vi "Get Parameters Configuration File Path.vi"(8 "error in":errorcluster, 11 "custom device ref":T1 format="%.0x") -> (0 "error out":errorcluster, 1 "MD5 checksum":string, 2 "parameters configuration file path":path, 3 "custom device ref out":T1 format="%.0x")   [LabVIEW 2024, in "AIM ARINC 429 Scripting.lvlib"]
doc: "Returns the <b>parameters configuration file path</b>. Systems configured in System Explorer must have a parameters configuration file. Scripted configurations do not require a parameters configuration file."
uses:
  AIM ARINC 429 Scripting.lvlib
  <vilib>/NI VeriStand/Custom Device API/Custom Device Item Ref.ctl
  Constants.vi
  <vilib>/NI VeriStand/Custom Device API/Get Item Property (Dependent File).vi
  <vilib>/NI VeriStand/Custom Device API/Custom Device API.lvlib
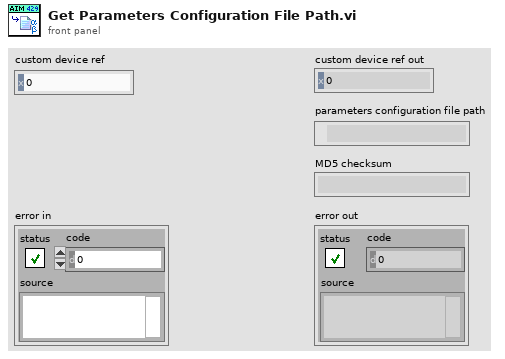
[diagram p1: front panel]
types:
  T1 = typedef "Custom Device API.lvlib/Custom Device Item Ref.ctl" = u64
  T2 = typedef "Custom Device API.lvlib/Dependent File Optional Info.ctl" = cluster{"Version":string, "RTDestination":path, "ForceDownload":bool, "SupportedTarget":string, "MD5":string}
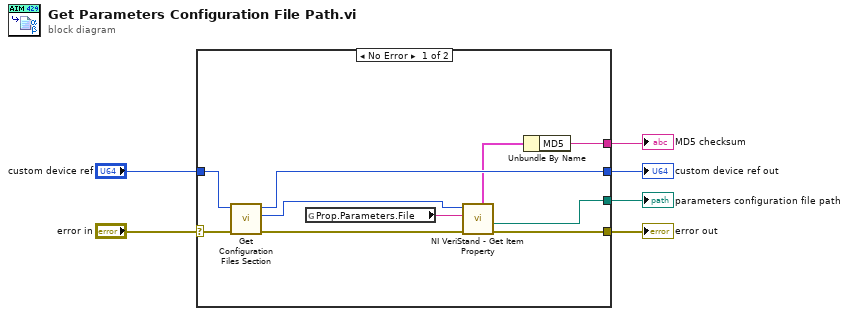
[diagram p0: block diagram]
diagram:
  n1 = case shown="No Error" "error in" {
    selector: "error in" -> [w11 w18]
    tunnel: "custom device ref" -> [w12 w17]
    tunnel: [w14 w18] -> w5
    tunnel: [w9 w17] -> w3
    tunnel: [w15 _] -> w2
    tunnel: [w7 _] -> w1
    frame No Error {
      n2 = call "Get Configuration Files Section.vi"("error in"=w11, "custom device ref"=w12) -> ("error out"=w10:errorcluster, "configuration files ref"=w13:T1, "custom device ref out"=w9:T1)  [unwired: 7 in]
      n3 = global read "Constants.vi" "Prop.Parameters.File"() -> (w16:string)
      n4 = call-poly <vilib>:"NI VeriStand - Get Item Property.vi"("error in (no error)"=w10, "Property Name"=w16, "Item Ref in"=w13) -> ("error out"=w14:errorcluster, "Path"=w15:path, "OptionalInfo"=w8:T2)  [unwired: 4 in, 2 out]
      n5 = Unbundle By Name(w8) -> ("MD5"=w7:string)
    }
    frame Error {
    }
  }
  "error out" <- w5
  "parameters configuration file path" <- w2
  "custom device ref out" <- w3
  "MD5 checksum" <- w1
